vi "Read Scan Size and Offset_Cypher.vi"(2 "Read in the string file":string) -> (5 "X Range (µm)":dbl, 6 "Y Range (µm)":dbl, 7 "X Offset (µm)":dbl, 8 "Y Offset (µm)":dbl)   [LabVIEW 2016]
uses:
  <vilib>/regexp/Match Regular Expression.xnode
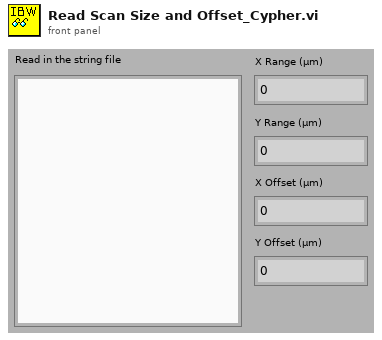
[diagram p1: front panel]
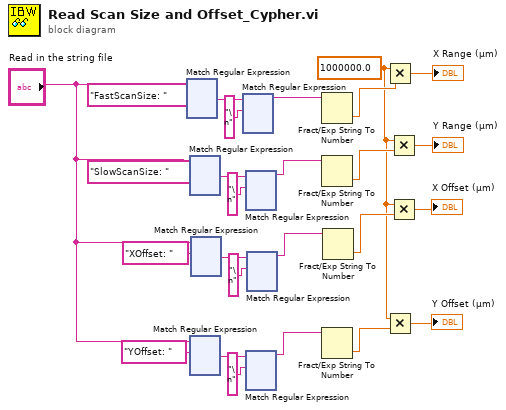
[diagram p0: block diagram]
diagram:
  w2 = 1000000.0 ("x")
  n1 = xnode "Match Regular Expression"("input string"="Read in the string file", "regular expression"="FastScanSize: ") -> ("after match"=w25:string)  [unwired: 2 in, 6 out]
  n2 = xnode "Match Regular Expression"("input string"="Read in the string file", "regular expression"="SlowScanSize: ") -> ("after match"=w21:string)  [unwired: 2 in, 6 out]
  n3 = xnode "Match Regular Expression"("input string"="Read in the string file", "regular expression"="YOffset: ") -> ("after match"=w6:string)  [unwired: 2 in, 6 out]
  n4 = xnode "Match Regular Expression"("input string"="Read in the string file", "regular expression"="XOffset: ") -> ("after match"=w17:string)  [unwired: 2 in, 6 out]
  n5 = xnode "Match Regular Expression"("input string"=w25, "regular expression"="\n") -> ("before match"=w23:string)  [unwired: 2 in, 6 out]
  n6 = xnode "Match Regular Expression"("input string"=w21, "regular expression"="\n") -> ("before match"=w19:string)  [unwired: 2 in, 6 out]
  n7 = xnode "Match Regular Expression"("input string"=w6, "regular expression"="\n") -> ("before match"=w8:string)  [unwired: 2 in, 6 out]
  n8 = xnode "Match Regular Expression"("input string"=w17, "regular expression"="\n") -> ("before match"=w11:string)  [unwired: 2 in, 6 out]
  n9 = Fract/Exp String To Number(string=w23) -> (number=w15:dbl)  [unwired: 3 in, 1 out]
  n10 = Fract/Exp String To Number(string=w19) -> (number=w13:dbl)  [unwired: 3 in, 1 out]
  n11 = Fract/Exp String To Number(string=w8) -> (number=w3:dbl)  [unwired: 3 in, 1 out]
  n12 = Fract/Exp String To Number(string=w11) -> (number=w10:dbl)  [unwired: 3 in, 1 out]
  n13 = Multiply(x=w2, y=w15) -> (x*y=→"X Range (µm)":dbl)
  n14 = Multiply(x=w2, y=w3) -> (x*y=→"Y Offset (µm)":dbl)
  n15 = Multiply(x=w2, y=w13) -> (x*y=→"Y Range (µm)":dbl)
  n16 = Multiply(x=w2, y=w10) -> (x*y=→"X Offset (µm)":dbl)
